vi "Real Outer Product.vi"(2 "Y Vector":dbl[](array[numeric]) format="%.2f", 3 "X Vector":dbl[](array[numeric]) format="%.2f") -> (0 "error":i32, 1 "Outer Product":T1)   [LabVIEW 2017, in "NI_AALBase.lvlib"]
doc: "Computes the outer product of <B>X Vector</B> and <B>Y Vector</B>. The data types you wire to the <B>X Vector</B> and <B>Y Vector</B> inputs determine the polymorphic instance to use."
uses:
  <vilib>/Analysis/NI_AALBase.lvlib
  <vilib>/Analysis/Matrix/Datatypes/RealMatrix.ctl
  <resource>/lvanlys.dll
  <vilib>/Analysis/Matrix/NI_Matrix.lvlib
panel:
  # "Outer Product"
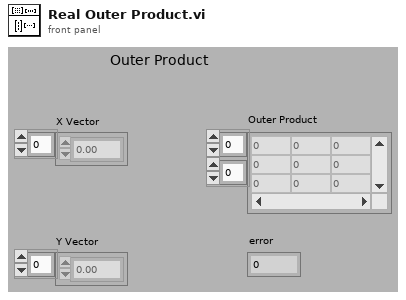
[diagram p1: front panel]
types:
  T1 = typedef "NI_Matrix.lvlib/RealMatrix.ctl" = dbl[][]
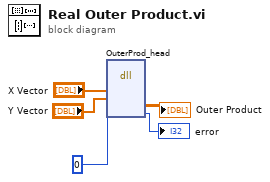
[diagram p0: block diagram]
diagram:
  n1 = dll-call lib="e:/builds/penguin/labview/branches/2017/dev/dist/resource/lvanlys.*" fn="OuterProd_head"("X Vector"="X Vector", "Y Vector"="Y Vector", 0) -> ("Outer Product"=→"Outer Product":T1, →"error":i32)  [unwired: 7 in, 2 out]
